vi "Flatten Names (String).vi"(0 "names in":string[](array[string]), 11 "error in (no error)":errorcluster) -> (4 "names out":string, 15 "error out":errorcluster)   [LabVIEW 2020, in "SLSC.lvlib"]
doc: "Converts an array of strings into a comma-delimited list of strings. If the array contains physical channel-style names with consecutive numeric suffixes, they will be collapsed into a colon-delimited range. Example: [\"Mod1\",\"Mod1/load0\",\"Mod1/capabilities\"] -> [\"Mod1,Mod1/load0,Mod1/capabilities\"]."
uses:
  <vilib>/SLSC/SLSC.lvlib
  nislsclvapi.dll
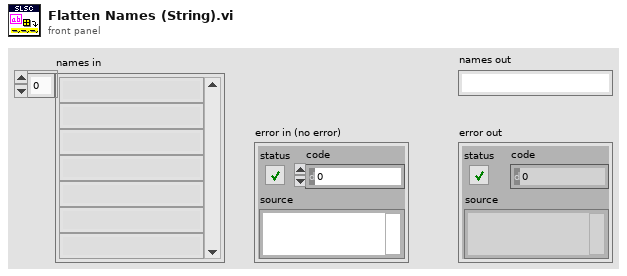
[diagram p1: front panel]
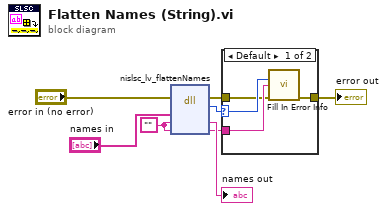
[diagram p0: block diagram]
diagram:
  w5 = ""
  n1 = dll-call lib="nislsclvapi.*" fn="nislsc_lv_flattenNames"(error in="error in (no error)", "namesIn"="names in", "namesOut"=w5, "extendedErrorInfo"=w5) -> (error out=w3:errorcluster, "return type"=w2:i32, "namesOut"=→"names out":string, "extendedErrorInfo"=w4:string)  [unwired: 3 in, 1 out]
  n2 = case shown="Default" w2 {
    selector: w2 -> [w12 _]
    tunnel: w4 -> [w11 _]
    tunnel: w3 -> [w10 w13]
    tunnel: [w9 w13] -> w1
    frame Default {
      n3 = call <vilib>:"Fill In Error Info.vi"("status code"=w12, "extended error info"=w11, "error in"=w10) -> ("error out"=w9:errorcluster)  [unwired: 12 in]
    }
    frame 0 {
    }
  }
  "error out" <- w1
